vi "Read Incoming Bytes.vi"(8 "error in (no error)":errorcluster, 9 "timeout (1000 ms)":i32=1000, 10 "bytes to read (100)":i32=100, 11 "LocalQueueConnection in":refnum<class "LocalQueueConnection.lvclass">) -> (0 "error out":errorcluster, 1 "timed out":bool, 2 "Bytes":u8[](array[numeric]) format="%08b", 3 "LocalQueueConnection":refnum<class "LocalQueueConnection.lvclass">, 4 "connected":bool)   [LabVIEW 2013, in "MQTT_Queue.lvlib" / "LocalQueueConnection.lvclass"]
uses:
  LocalQueueConnection.lvclass
  LocalQueueConnection.lvclass/LocalQueueConnection.ctl
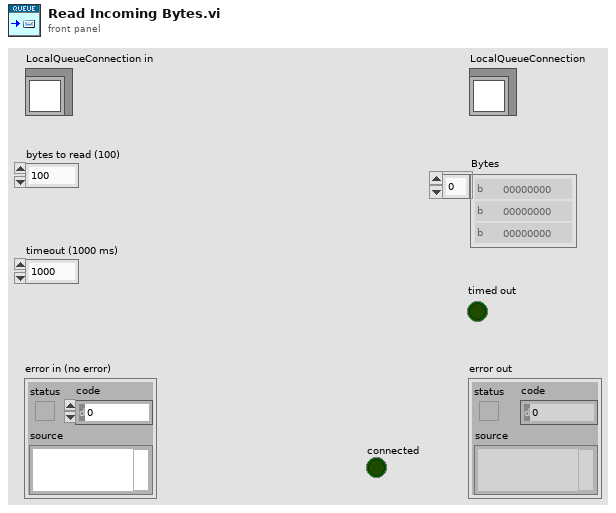
[diagram p1: front panel]
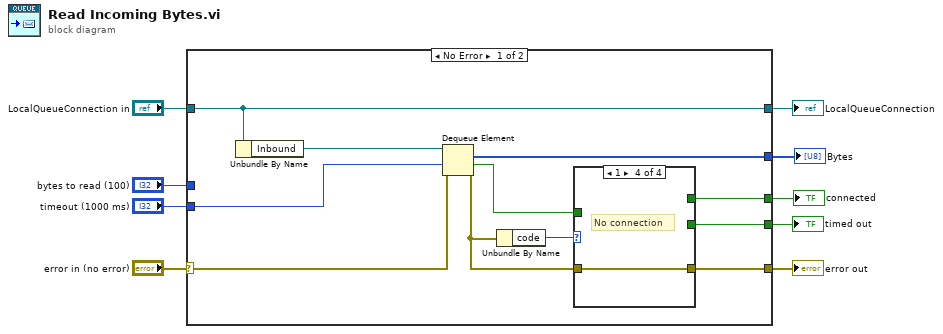
[diagram p0: block diagram]
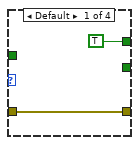
[diagram p2: hidden frame]
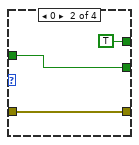
[diagram p3: hidden frame]
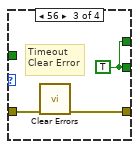
[diagram p4: hidden frame]
diagram:
  n1 = case shown="No Error" "error in (no error)" {
    selector: "error in (no error)" -> [w14 w31]
    tunnel: [w17 w31] -> w8
    tunnel: [w18 w30] -> w6
    tunnel: "LocalQueueConnection in" -> [w18 w30]
    tunnel: [w13 _] -> w5
    tunnel: "bytes to read (100)" -> [_ _]
    tunnel: "timeout (1000 ms)" -> [w12 _]
    tunnel: [w19 _] -> w2
    tunnel: [w16 _] -> w1
    frame No Error {
      n2 = Unbundle By Name(w18) -> ("Inbound"=w15:refnum<queue>)
      n3 = Dequeue Element(queue=w15, timeout in ms (-1)=w12, error in (no error)=w14) -> (element=w13:u8[], timed out?=w10:bool, error out=w11:errorcluster)  [unwired: 1 out]
      n4 = Unbundle By Name(w11) -> ("code"=w20:i32)
      n5 = case shown="1" w20 {
        tunnel: [w22 w25 w28 w29] -> w17
        tunnel: w11 -> [w22 w25 w27 w29]
        tunnel: [_ w23 w26 _] -> w19
        tunnel: [TRUE TRUE w26 _] -> w16
        tunnel: w10 -> [_ w23 _ _]
        frame Default {
        }
        frame 0 {
        }
        frame 56 {
          w26 = TRUE
          # "Timeout\nClear Error"
          n6 = call <vilib>:"Clear Errors.vi"("error in (no error)"=w27) -> ("error out"=w28:errorcluster)  [unwired: 6 in]
        }
        frame 1 {
          # "No connection"
        }
      }
    }
    frame Error {
    }
  }
  "error out" <- w8
  "LocalQueueConnection" <- w6
  "Bytes" <- w5
  "timed out" <- w2
  "connected" <- w1
